vi "FilterWindVane.vi"(9 "Queue timeout (ms)":i32=200, 10 "NotifierReff 2":T2, 11 "Wind Vane Queue Cluster":T1) -> ()   [LabVIEW 2013]
doc: "Performs and filtering that we want (default is no filtering) and writes the data to the notifier. If no data is in the queue this VI times out after 'Queue timeout (ms)' has passed and nothing is written to the notifier.\n\nEric Schneider, March 2014"
uses:
  Data/TypeDefs/Notifiers.ctl
  Data/TypeDefs/UTM Location.ctl
  Data/TypeDefs/Sail Set Suggestions.ctl
  Data/TypeDefs/Rudder Set Suggestions.ctl
  Data/TypeDefs/OverrideInformation.ctl
  Data/TypeDefs/OverrideMode.ctl
  Data/TypeDefs/MotorSetup.ctl
  Data/TypeDefs/DynamixelSetupInfo.ctl
  Data/TypeDefs/AirmarStatus.ctl
  Data/TypeDefs/HardwareOnline.ctl
  Data/TypeDefs/WindData Queue Cluster.ctl
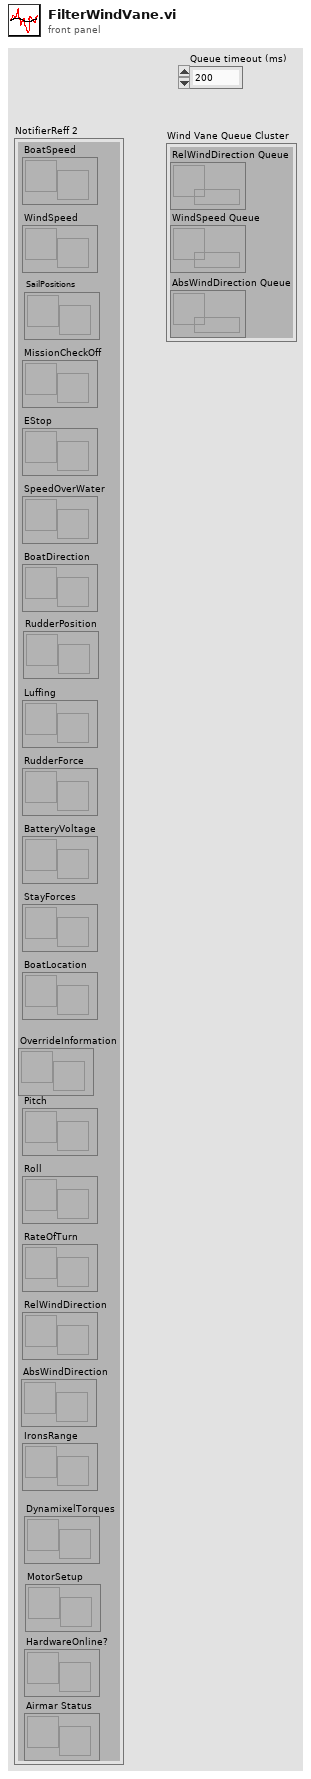
[diagram p1: front panel]
types:
  T1 = typedef "WindData Queue Cluster.ctl" = cluster{"RelWindDirection Queue":refnum<queue>, "WindSpeed Queue":refnum<queue>, "AbsWindDirection Queue":refnum<queue>}
  T2 = typedef "Notifiers.ctl" = cluster{"BoatSpeed":refnum<notifier>, "WindSpeed":refnum<notifier>, "MissionCheckOff":refnum<notifier>, "EStop":refnum<notifier>, "SpeedOverWater":refnum<notifier>, "BoatDirection":refnum<notifier>, "Luffing":refnum<notifier>, "RudderForce":refnum<notifier>, "BatteryVoltage":refnum<notifier>, "StayForces":refnum<notifier>, "BoatLocation":refnum<notifier>, "Pitch":refnum<notifier>, "Roll":refnum<notifier>, "RateOfTurn":refnum<notifier>, "RelWindDirection":refnum<notifier>, "SailPositions":refnum<notifier>, "RudderPosition":refnum<notifier>, "IronsRange":refnum<notifier>, "AbsWindDirection":refnum<notifier>, "OverrideInformation":refnum<notifier>, "DynamixelTorques":refnum<notifier>, "MotorSetup":refnum<notifier>, "Airmar Status":refnum<notifier>, "HardwareOnline?":refnum<notifier>}
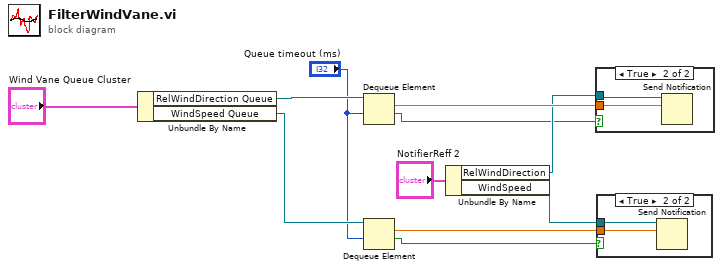
[diagram p0: block diagram]
diagram:
  n1 = Unbundle By Name("Wind Vane Queue Cluster") -> ("RelWindDirection Queue"=w9:refnum<queue>, "WindSpeed Queue"=w8:refnum<queue>)
  n2 = Dequeue Element(queue=w9, timeout in ms (-1)="Queue timeout (ms)") -> (element=w11:dbl, timed out?=w2:bool)  [unwired: 1 in, 2 out]
  n3 = Dequeue Element(queue=w8, timeout in ms (-1)="Queue timeout (ms)") -> (element=w4:dbl, timed out?=w1:bool)  [unwired: 1 in, 2 out]
  n4 = Unbundle By Name("NotifierReff 2") -> ("RelWindDirection"=w6:refnum<notifier>, "WindSpeed"=w5:refnum<notifier>)
  n5 = case shown="True" w2 {
    tunnel: w11 -> [_ w13]
    tunnel: w6 -> [_ w12]
    frame False {
    }
    frame True {
      n6 = Send Notification(notification=w13, notifier=w12) -> ()  [unwired: 1 in, 2 out]
    }
  }
  n7 = case shown="True" w1 {
    tunnel: w5 -> [_ w15]
    tunnel: w4 -> [_ w14]
    frame False {
    }
    frame True {
      n8 = Send Notification(notification=w14, notifier=w15) -> ()  [unwired: 1 in, 2 out]
    }
  }
